vi "create_ir.vi"(8 "error in (no error)":errorcluster, 10 "device_name":string="CPU", 11 "xml_file":path) -> (0 "error out":errorcluster, 3 "OvEngineStruct":u64)   [LabVIEW 2023]
uses:
  openvino_vi_wrapper.dll
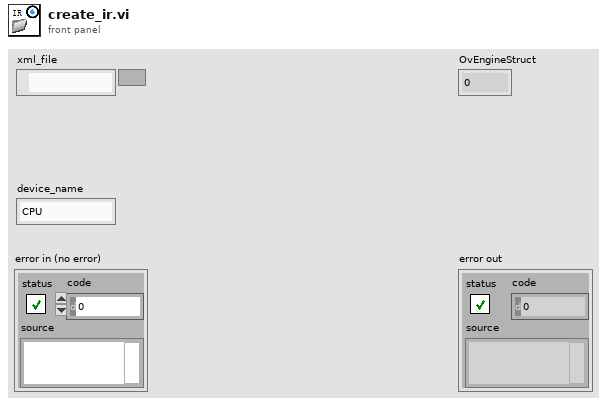
[diagram p1: front panel]
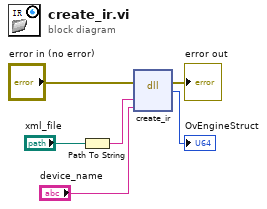
[diagram p0: block diagram]
diagram:
  n1 = Path To String(path="xml_file") -> (string=w5:string)
  n2 = dll-call lib="C:/Users/NUC/Desktop/LabVIEW_OpenVINO_Dll/yolov8_openvino_opensource/openvino_vi_wrapper/openvino_vi_wrapper.dll" fn="create_ir"(error in="error in (no error)", "xmlFile"=w5, "device_name"="device_name") -> (error out=→"error out":errorcluster, "InferEngineStruct"=→"OvEngineStruct":u64)  [unwired: 4 in, 1 out]
